vi "Access Class Directory.vi"(8 "error in":errorcluster, 11 "Config in":refnum<class "Config.lvclass">) -> (0 "error out":errorcluster, 1 "Class Names":string[](array[string]), 2 "Class Paths":path[](array[path]), 3 "Config out":refnum<class "Config.lvclass">)   [LabVIEW 2023, in "Config.lvlib" / "Config.lvclass"]
uses:
  Config.lvclass
  <vilib>/Utility/LVLibp/NI_PackedLibraryUtility.lvlib
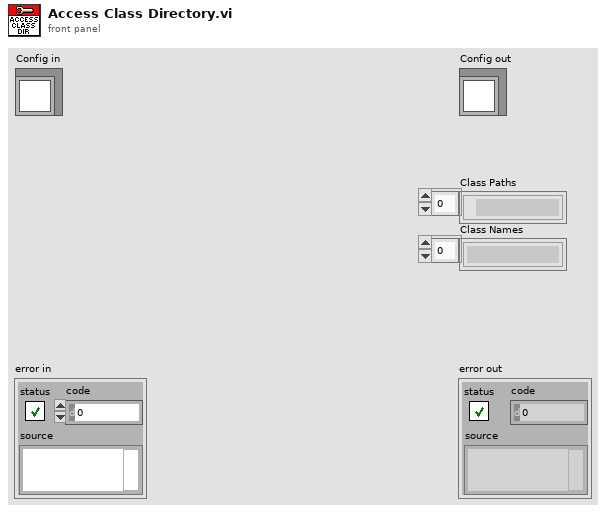
[diagram p1: front panel]
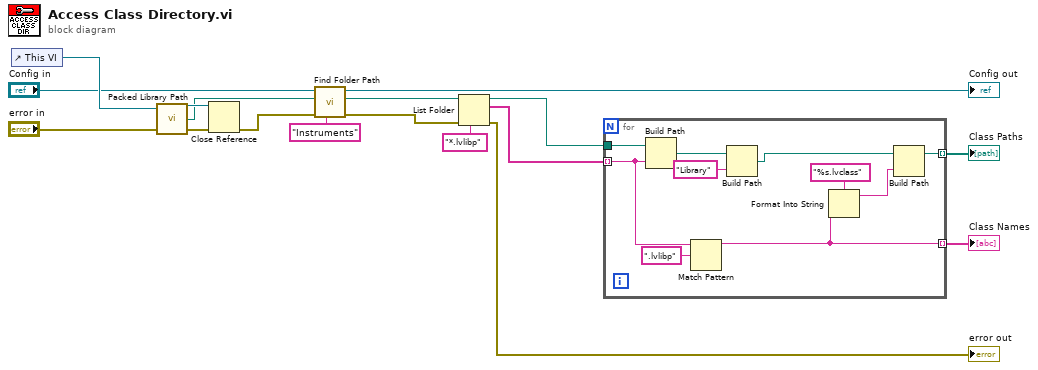
[diagram p0: block diagram]
diagram:
  n1 = control-ref of="This VI"() -> (w15:refnum<vi>)
  n2 = call <vilib>:"Packed Library Path.vi"("error in (no error)"="error in", "vi reference"=w15) -> ("error out"=w16:errorcluster, "packed library path"=w1:path, "vi reference out"=w17:refnum<vi>)  [unwired: 1 in]
  n3 = Close Reference(reference=w17, error in (no error)=w16) -> (error out=w6:errorcluster)
  n4 = call "Find Folder Path.vi"("File Name\nwith extension"="Instruments" ("File Name\nwith extension"), "error in"=w6, "Path\n(Empty at top level)"=w1, "Config in"="Config in") -> ("error out"=w3:errorcluster, "File Path Control"=w5:path, "Config out"=→"Config out":refnum<class "Config.lvclass">)  [unwired: 5 in]
  n5 = List Folder(path=w5, pattern="*.lvlibp", error in=w3) -> (path out=w12:path, filenames=w11:string[], error out=→"error out":errorcluster)  [unwired: 1 in, 1 out]
  n6 = for {
    tunnel: w12 -> [w27]
    tunnel: w11 -> [w24] mode=indexing
    tunnel: [w25] -> w10 mode=indexing
    tunnel: [w22] -> w9 mode=indexing
    n7 = Build Path(base path=w27, name or relative path=w24) -> (appended path=w20:path)
    n8 = Match Pattern(string=w24, regular expression=".lvlibp") -> (before substring=w22:string)  [unwired: 1 in, 3 out]
    n9 = Build Path(base path=w20, name or relative path="Library") -> (appended path=w18:path)
    n10 = Format Into String(format string="%s.lvclass", w22) -> (resulting string=w21:string)  [unwired: 2 in, 1 out]
    n11 = Build Path(base path=w18, name or relative path=w21) -> (appended path=w25:path)
  }
  "Class Paths" <- w10
  "Class Names" <- w9
